vi "Draw Animation.vi"(4 "3D Scene Ref":refnum<vi>, 7 "3D Comet Property":T4={"General Property"={"Plot Name"="", "Coordinate System"=enum."Cartesian", "Opacity"=0.0}, "Projection Property"={"Draw XY"=FALSE, "Draw YZ"=FALSE, "Draw XZ"=FALSE}, "Plot Property"={"Sprite Type"=enum."Empty Square", "Point Size"=0.0, "Point Color"=0, "Line Style"=enum."None", "Line Width"=0.0, "Line Color"=0, "Antialiasing"=FALSE}, "Comet Property"={"Body length"=0.0}}, 8 "error in (no error)":errorcluster, 9 "Actual Transform In":T7, 10 "Plot Representation In":T1, 11 "Plot Object In":refnum<vi>) -> (0 "error out":errorcluster, 1 "Actual Transform Out":T7, 2 "Plot Representation Out":T1, 3 "Plot Object Out":refnum<vi>)   [LabVIEW 2020, in "3D Comet.lvclass"]
uses:
  <vilib>/Math Plots/3D Math Plots/3D Comet/3D Comet/3D Comet.lvclass
  <vilib>/Math Plots/3D Math Plots/3D Plot/3D Plot/Typedef/Actual Transform.ctl
  <vilib>/Math Plots/3D Math Plots/3D Plot/3D Plot/Typedef/Range Clusters.ctl
  <vilib>/Math Plots/3D Math Plots/3D Plot/3D Plot/Typedef/Plot Representation.ctl
  <vilib>/Math Plots/3D Math Plots/3D Plot/3D Plot/Typedef/Mesh Data.ctl
  <vilib>/Math Plots/3D Math Plots/3D Comet/3D Comet/Typedef/3D Comet Property.ctl
  <vilib>/Math Plots/3D Math Plots/3D Plot/3D Plot/Typedef/Sprite Type.ctl
  <vilib>/Math Plots/3D Math Plots/3D Plot/3D Plot/Typedef/Line Type.ctl
  <vilib>/picture/3D Picture Control/NI_3D Picture Control.lvlib
  <vilib>/Math Plots/3D Math Plots/3D Plot/3D Plot/3D Plot.lvclass
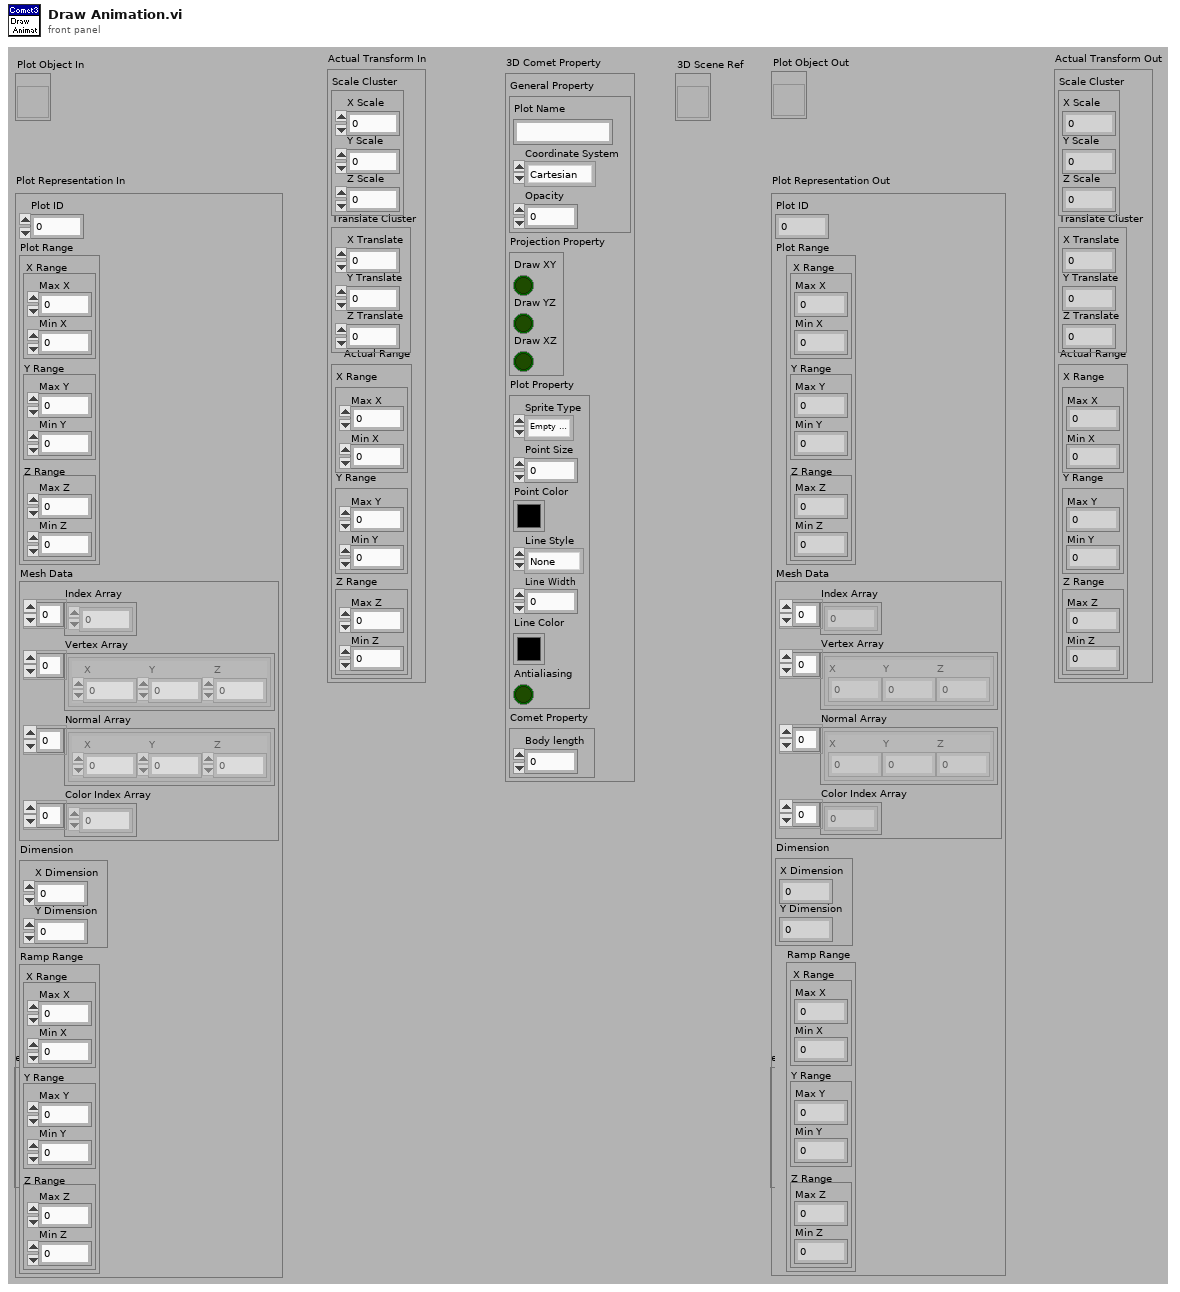
[diagram p1: front panel]
types:
  T1 = typedef "3D Plot.lvclass/Plot Representation.ctl" = cluster{"Plot ID":i32, "Plot Range":T2, "Mesh Data":T3, "Dimension":cluster{"X Dimension":i32, "Y Dimension":i32}, "Ramp Range":T2}
  T2 = typedef "3D Plot.lvclass/Range Clusters.ctl" = cluster{"X Range":cluster{"Max X":sgl, "Min X":sgl}, "Y Range":cluster{"Max Y":sgl, "Min Y":sgl}, "Z Range":cluster{"Max Z":sgl, "Min Z":sgl}}
  T3 = typedef "3D Plot.lvclass/Mesh Data.ctl" = cluster{"Index Array":u32[], "Vertex Array":cluster{"X":sgl, "Y":sgl, "Z":sgl}[], "Normal Array":cluster{"X":sgl, "Y":sgl, "Z":sgl}[], "Color Index Array":i32[]}
  T4 = typedef "3D Comet.lvclass/3D Comet Property.ctl" = cluster{"General Property":cluster{"Plot Name":string, "Coordinate System":enum16{"Cartesian", "Cylindrical", "Spherical"}, "Opacity":sgl}, "Projection Property":cluster{"Draw XY":bool, "Draw YZ":bool, "Draw XZ":bool}, "Plot Property":cluster{"Sprite Type":T5, "Point Size":sgl, "Point Color":u32, "Line Style":T6, "Line Width":sgl, "Line Color":u32, "Antialiasing":bool}, "Comet Property":cluster{"Body length":sgl}}
  T5 = typedef "3D Plot.lvclass/Sprite Type.ctl" = enum16{"None", "Empty Square", "Solid Square", "Empty Diamond", "Solid Diamond", "Empty Circle", "Solid Circle", "Asterisk", "Bold X", "Wireframe Sphere", "Solid Sphere", "Wireframe Cube", "Solid Cube"}
  T6 = typedef "3D Plot.lvclass/Line Type.ctl" = enum16{"None", "Solid", "Dash", "Dot", "Dash Dot"}
  T7 = typedef "3D Plot.lvclass/Actual Transform.ctl" = cluster{"Scale Cluster":cluster{"X Scale":sgl, "Y Scale":sgl, "Z Scale":sgl}, "Translate Cluster":cluster{"X Translate":sgl, "Y Translate":sgl, "Z Translate":sgl}, "Actual Range":T2}
  T8 = cluster{"X Scale":sgl, "Y Scale":sgl, "Z Scale":sgl}
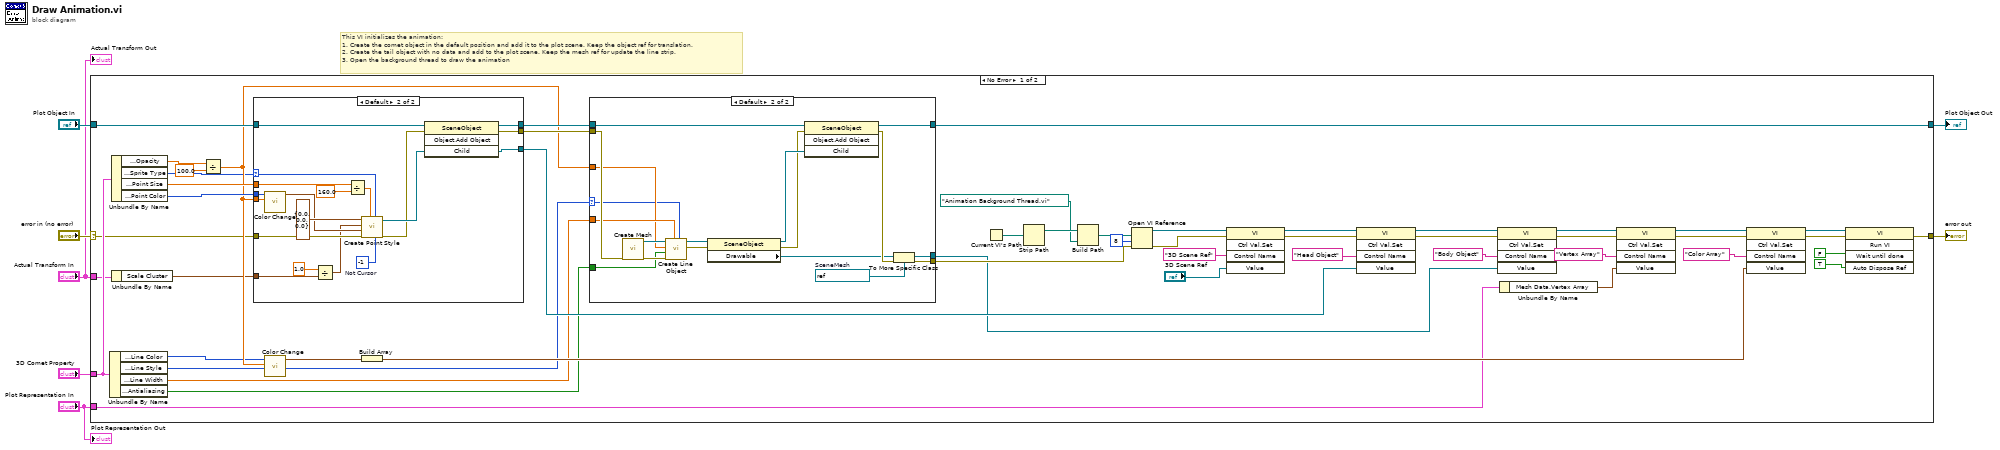
[diagram p0: block diagram]
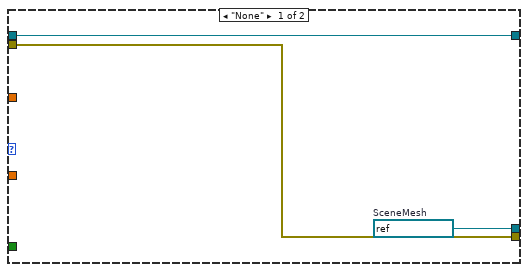
[diagram p2: hidden frame]
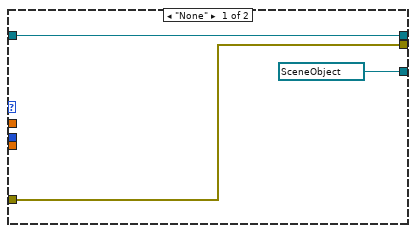
[diagram p3: hidden frame]
diagram:
  # "This VI initializes the animation:\n1. Create the comet object in the default position and add it to the plot scene. Keep the object ref for translation.\n2. Create the tail object with no data and add to the plot scene. Keep the mesh ref for update the line strip.\n3. Open the background thread to draw the animation"
  n1 = case shown="No Error" "error in (no error)" {
    selector: "error in (no error)" -> [w13 w102]
    tunnel: [w54 w103] -> w7
    tunnel: "Plot Object In" -> [w28 w103]
    tunnel: "Plot Representation In" -> [w27 _]
    tunnel: "3D Comet Property" -> [w20 _]
    tunnel: [w8 w102] -> w1
    tunnel: "Actual Transform In" -> [w12 _]
    frame No Error {
      n2 = Unbundle By Name(w20) -> ("Plot Property.Line Color"=w16:u32, "Plot Property.Line Style"=w17:T6, "Plot Property.Line Width"=w18:sgl, "Plot Property.Antialiasing"=w19:bool)
      n3 = Unbundle By Name(w20) -> ("General Property.Opacity"=w58:sgl, "Plot Property.Sprite Type"=w21:T5, "Plot Property.Point Size"=w26:sgl, "Plot Property.Point Color"=w56:u32)
      n4 = Unbundle By Name(w12) -> ("Scale Cluster"=w11:T8)
      n5 = Divide(x=w58, y=sgl 100.0) -> (x/y=w22:sgl)
      n6 = case shown="Default" w21 {
        selector: w21 -> [_ w86]
        tunnel: w56 -> [_ w101]
        tunnel: [w81 w100] -> w55
        tunnel: [refnum<vi> refnum ("Child") w99] -> w48
        tunnel: w28 -> [w81 w98]
        tunnel: w13 -> [w80 w93]
        tunnel: w26 -> [_ w91]
        tunnel: [w80 w88] -> w23
        tunnel: w22 -> [_ w87]
        tunnel: w11 -> [_ w84]
        frame "None" {
        }
        frame Default {
          w89 = -1  # Not Cursor
          n7 = call <vilib>:"Color Change.vi"("Alpha"=w87, "Color"=w101) -> ("RGBA"=w96:cluster{"R":sgl, "G":sgl, "B":sgl, "A":sgl})  [unwired: 9 out]
          n8 = Divide(x=sgl 1.0, y=w84) -> (x/y=w83:T8)
          n9 = Divide(x=w91, y=sgl 160.0) -> (x/y=w90:sgl)
          n10 = call <vilib>:"Create Point Style.vi"("Cursor ID"=w89, "Sprite Type"=w86, "Size"=w90, "error in (no error)"=w93, "RGBA"=w96, "Scale"=w83, "Position"=cluster{"X":sgl, "Y":sgl, "Z":sgl} {"X"=0.0, "Y"=0.0, "Z"=0.0} ("3D Point")) -> ("error out"=w94:errorcluster, "Scene:New Object"=w95:refnum<vi>)  [unwired: 1 in, 2 out]
          n11 = invoke class="SceneObject" method="Object.Add Object"(reference=w98, error in=w94, "Child"=w95) -> (reference out=w100:refnum<vi>, error out=w88:errorcluster, "Child"=w99:refnum<vi>)  [unwired: 1 in, 1 out]
        }
      }
      n12 = call <vilib>:"Color Change.vi"("Alpha"=w22, "Color"=w16) -> ("RGBA"=w46:cluster{"R":sgl, "G":sgl, "B":sgl, "A":sgl})  [unwired: 9 out]
      n13 = Build Array(w46) -> (w45:cluster{"R":sgl, "G":sgl, "B":sgl, "A":sgl}[])
      n14 = case shown="Default" w17 {
        selector: w17 -> [_ w62]
        tunnel: w55 -> [w61 w79]
        tunnel: [w61 w78] -> w54
        tunnel: [w59 w75] -> w49
        tunnel: [w60 w74] -> w47
        tunnel: w23 -> [w59 w72]
        tunnel: w18 -> [_ w70]
        tunnel: w22 -> [_ w69]
        tunnel: w19 -> [_ w68]
        frame "None" {
          w60 = refnum<vi> refnum  # SceneMesh
        }
        frame Default {
          w77 = refnum<vi> refnum  # SceneMesh
          n15 = call <vilib>:"Create Mesh.vi"("error in (no error)"=w72) -> ("error out"=w71:errorcluster, "New Mesh Refnum"=w73:refnum<vi>)  [unwired: 9 out]
          n16 = call <vilib>:"Create Line Object.vi"("Line Style"=w62, "Line Width"=w70, "error in (no error)"=w71, "Antialiasing"=w68, "Alpha"=w69, "Mesh Ref In"=w73) -> ("error out"=w64:errorcluster, "Object Ref Out"=w67:refnum<vi>)  [unwired: 4 out]
          n17 = property class="SceneObject"(reference=w67, error in=w64) -> (reference out=w66:refnum<vi>, error out=w63:errorcluster, "Drawable"=w65:refnum<vi>)
          n18 = invoke class="SceneObject" method="Object.Add Object"(reference=w79, error in=w63, "Child"=w66) -> (reference out=w78:refnum<vi>, error out=w76:errorcluster)  [unwired: 1 in, 2 out]
          n19 = To More Specific Class(target class=w77, reference=w65, error in=w76) -> (specific class reference=w74:refnum<vi>, error out=w75:errorcluster)
        }
      }
      n20 = Current VI's Path() -> (path=w53:path)
      n21 = Strip Path(path=w53) -> (stripped path=w52:path)  [unwired: 1 out]
      n22 = Build Path(base path=w52, name or relative path=path "Animation Background Thread.vi") -> (appended path=w50:path)
      n23 = Open VI Reference(vi path=w50, options=8, error in (no error)=w49) -> (vi reference=w14:refnum<vi>, error out=w10:errorcluster)  [unwired: 1 in, 2 out]
      n24 = invoke class="VI" method="Ctrl Val.Set"(reference=w14, error in=w10, "Control Name"="3D Scene Ref", "Value"="3D Scene Ref") -> (reference out=w25:refnum<vi>, error out=w24:errorcluster)  [unwired: 1 in, 3 out]
      n25 = invoke class="VI" method="Ctrl Val.Set"(reference=w25, error in=w24, "Control Name"="Head Object", "Value"=w48) -> (reference out=w40:refnum<vi>, error out=w9:errorcluster)  [unwired: 1 in, 3 out]
      n26 = invoke class="VI" method="Ctrl Val.Set"(reference=w40, error in=w9, "Control Name"="Body Object", "Value"=w47) -> (reference out=w38:refnum<vi>, error out=w37:errorcluster)  [unwired: 1 in, 3 out]
      n27 = Unbundle By Name(w27) -> ("Mesh Data.Vertex Array"=w33:cluster{"X":sgl, "Y":sgl, "Z":sgl}[])
      n28 = invoke class="VI" method="Ctrl Val.Set"(reference=w38, error in=w37, "Control Name"="Vertex Array", "Value"=w33) -> (reference out=w30:refnum<vi>, error out=w29:errorcluster)  [unwired: 1 in, 3 out]
      n29 = invoke class="VI" method="Ctrl Val.Set"(reference=w30, error in=w29, "Control Name"="Color Array", "Value"=w45) -> (reference out=w36:refnum<vi>, error out=w35:errorcluster)  [unwired: 1 in, 3 out]
      n30 = invoke class="VI" method="Run VI"(reference=w36, error in=w35, "Wait until done"=FALSE ("Wait Until Done"), "Auto Dispose Ref"=TRUE ("Auto Dispose Reference")) -> (error out=w8:errorcluster)  [unwired: 1 in, 4 out]
    }
    frame Error {
    }
  }
  "Plot Object Out" <- w7
  "error out" <- w1
  "Actual Transform Out" <- "Actual Transform In"
  "Plot Representation Out" <- "Plot Representation In"
